vi "FTW-STR-Split-Comma.vi"(5 "Delimited String":string) -> (6 "Array of Strings":string[](array[string]))   [LabVIEW 2015]
panel:
  # "Inputs"
  # "Outputs"
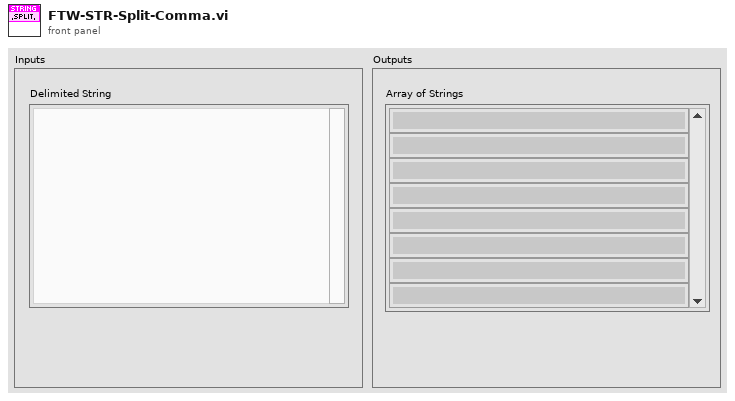
[diagram p1: front panel]
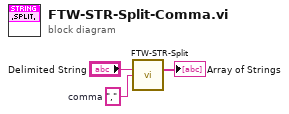
[diagram p0: block diagram]
diagram:
  w1 = ","  # comma
  n1 = call "FTW-STR-Split.vi"("Delimited String"="Delimited String", "Delimiter"=w1) -> ("Array of Strings"=→"Array of Strings":string[])  [unwired: 13 in]
